vi "TSM SSC Digital Configure Time Set Compare Edge Per-Site.vi"(0 "Digital TSM In":T1, 5 "time set":string caption="Time Set", 7 "Per-Site Compare Strobe (s)":dbl[](array[numeric]), 11 "error in":errorcluster) -> (4 "Digital TSM Out":T1, 15 "error out":errorcluster)   [LabVIEW 2019]
doc: "Configures the strobe edge time for the specified pins. Use this function to modify time set values after applying a timing sheet with the niDigital Apply Levels and Timing VI, or to create time sets programmatically without the use of timing sheets. This function does not modify the timing sheet file or the timing sheet contents that will be used in future calls to niDigital Apply Levels and Timing; it only affects the values of the current timing context."
uses:
  TSM/TSM SSC Digital.ctl
  <vilib>/NI_TestStand_SemiconductorModule/NI_TestStand_Semiconductor_Module.lvlibp/PinMap/Digital Pattern/PinQueryContext/DigitalPatternPinQueryContext.lvclass
  SSC Digital/SSC Digital.ctl
  9364476d-38f7-4630-a1cb-0fa518ee1b44.vi
  Shared SubVIs/Site List to Site Numbers.vi
  Shared SubVIs/Channel List to Pins.vi
  Shared SubVIs/Trim Whitespace [Inlined].vi
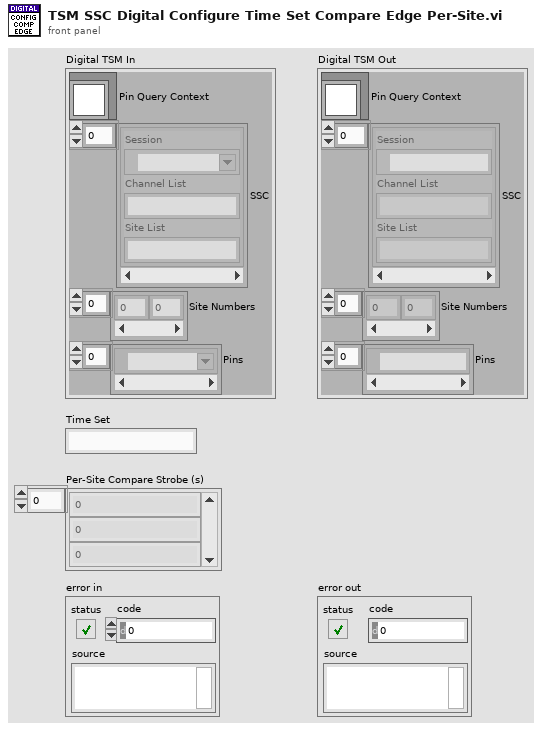
[diagram p1: front panel]
types:
  T1 = typedef "TSM SSC Digital.ctl" = cluster{"Pin Query Context":refnum<class "DigitalPatternPinQueryContext.lvclass">, "SSC":T2[], "Site Numbers":i32[], "Pins":tag[]}
  T2 = typedef "SSC Digital.ctl" = cluster{"Session":refnum<k15>, "Channel List":string, "Site List":string}
  T3 = typedef "Digital 2D Location.ctl" = cluster{"Row":i32, "Col":i32}
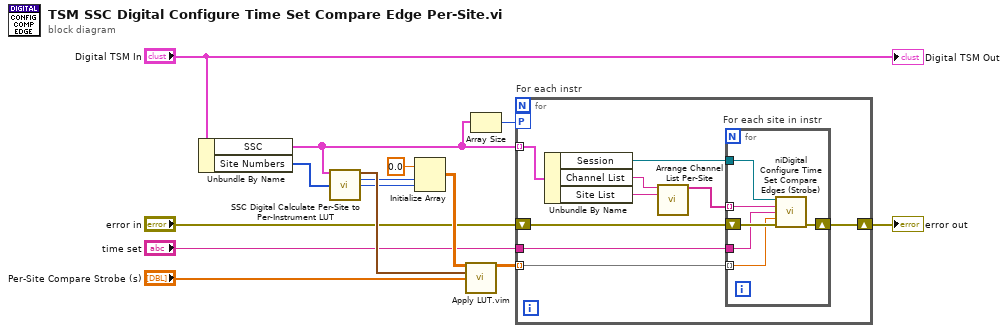
[diagram p0: block diagram]
diagram:
  n1 = Unbundle By Name("Digital TSM In") -> ("SSC"=w6:T2[], "Site Numbers"=w11:i32[])
  n2 = call "SSC Digital Calculate Per-Site to Per-Instrument LUT.vi"("Digital SSC In"=w6, "Sites"=w11) -> ("Per-Site to Per-Instrument LUT"=w12:T3[], "Instrument Count"=w9:i32, "Max Sites on Instrument"=w8:i32)  [unwired: 11 in]
  n3 = Initialize Array(0.0 ("element"), w9, w8) -> (w14:dbl[][])
  n4 = call "Apply LUT.vim"("Initialized Array"=w14, "LUT"=w12, "Results to Apply LUT to"="Per-Site Compare Strobe (s)") -> ("Array Out"=w10:dbl[][])  [unwired: 12 in]
  n5 = Array Size(array=w6) -> (size(s)=w7:i32)
  n6 = for "For each instr" {
    tunnel: "time set" -> [w15]
    workers-P: w7 -> [_]
    tunnel: w6 -> [w20] mode=indexing
    tunnel: w10 -> [w17] mode=indexing
    shift-right: [w22] -> w3
    shift-left: "error in" -> [w23]
    n7 = Unbundle By Name(w20) -> ("Session"=w16:refnum<k15>, "Channel List"=w19:string, "Site List"=w18:string)
    n8 = call "Arrange Channel List Per-Site.vi"("Channel List String"=w19, "Site List String"=w18) -> ("Channel List Array"=w21:string[])  [unwired: 11 in, 2 out]
    n9 = for "For each site in instr" {
      tunnel: w21 -> [w26] mode=indexing
      shift-right: [w29] -> w22
      shift-left: w23 -> [w28]
      tunnel: w17 -> [w24] mode=indexing
      tunnel: w16 -> [w27]
      tunnel: w15 -> [w25]
      n10 = call <instrlib>:"niDigital Configure Time Set Compare Edges (Strobe).vi"("instrument handle"=w27, "pin list"=w26, "edge set"=w25, "compare strobe (s)"=w24, "error in"=w28) -> ("error out"=w29:errorcluster)  [unwired: 9 in, 1 out]
    }
  }
  "error out" <- w3
  "Digital TSM Out" <- "Digital TSM In"
